vi "题目1.vi"() -> ()   [LabVIEW 2017]
panel:
  out "波形图表 2":dbl(graph)
  out "波形图表":dbl[](graph)
  in  "滑动杆 2":dbl(slide) scale=0.0..10.0
  in  "滑动杆":dbl(slide) scale=0.0..10.0
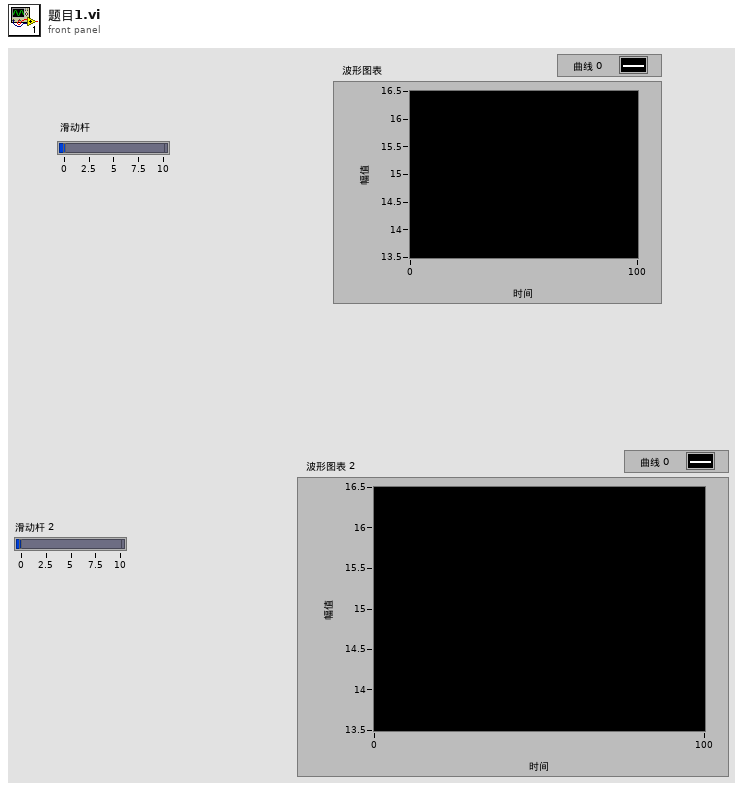
[diagram p1: front panel]
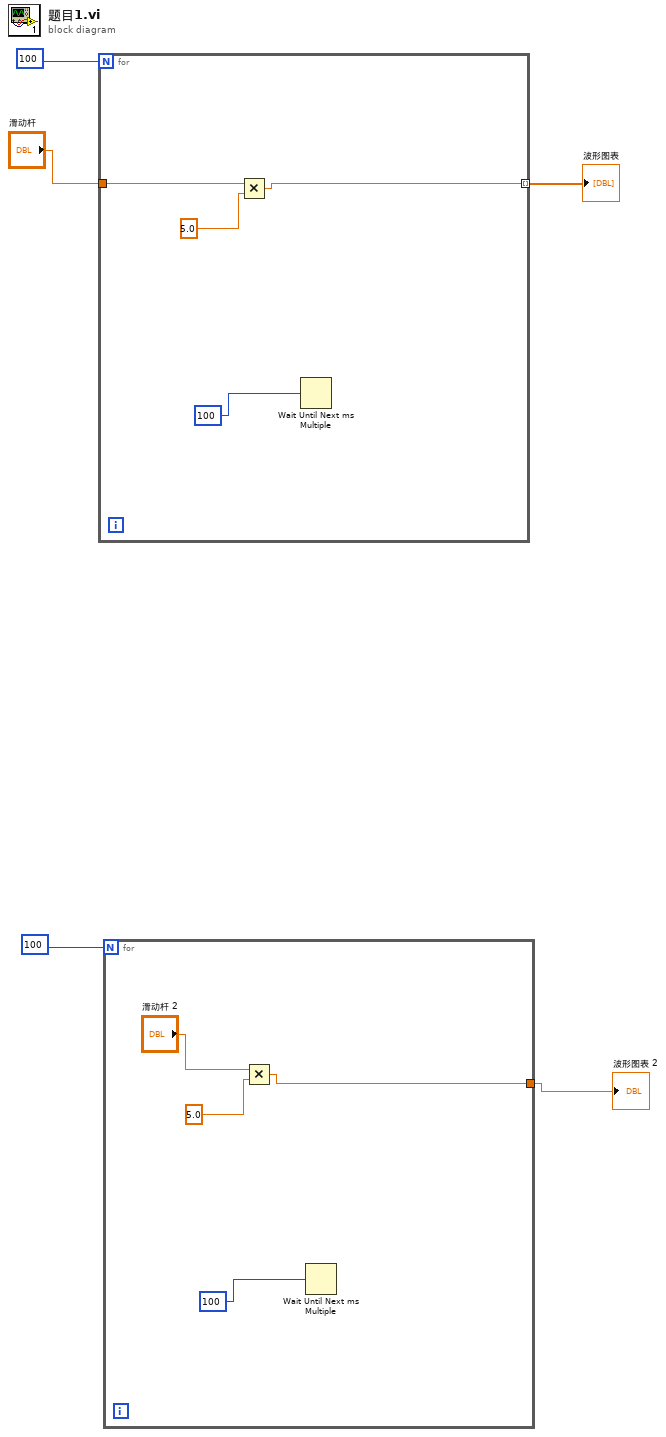
[diagram p0: block diagram]
diagram:
  n1 = for {
    N: 100 -> [_]
    tunnel: "滑动杆" -> [w8]
    tunnel: [w6] -> w2 mode=indexing
    n2 = Multiply(x=w8, y=5.0) -> (x*y=w6:dbl)
    n3 = Wait Until Next ms Multiple(millisecond multiple=100) -> ()  [unwired: 1 out]
  }
  "波形图表" <- w2
  n4 = for {
    N: 100 -> [_]
    tunnel: [w10] -> w1
    n5 = Multiply(x="滑动杆 2", y=5.0) -> (x*y=w10:dbl)
    n6 = Wait Until Next ms Multiple(millisecond multiple=100) -> ()  [unwired: 1 out]
  }
  "波形图表 2" <- w1
